vi "Get Kalman Filter State.vi"(11 "Kalman Filter In":T2) -> (0 "Predicted Covariance":T1, 1 "Predicted State":T1, 2 "Current Covariance":T1, 3 "Current State":T1)   [LabVIEW 2020]
uses:
  ctl/Kalman Filter Instance.ctl
  <vilib>/Analysis/Matrix/Datatypes/RealMatrix.ctl
  ctl/Dynamical System Matrices.ctl
  <vilib>/Analysis/Matrix/NI_Matrix.lvlib
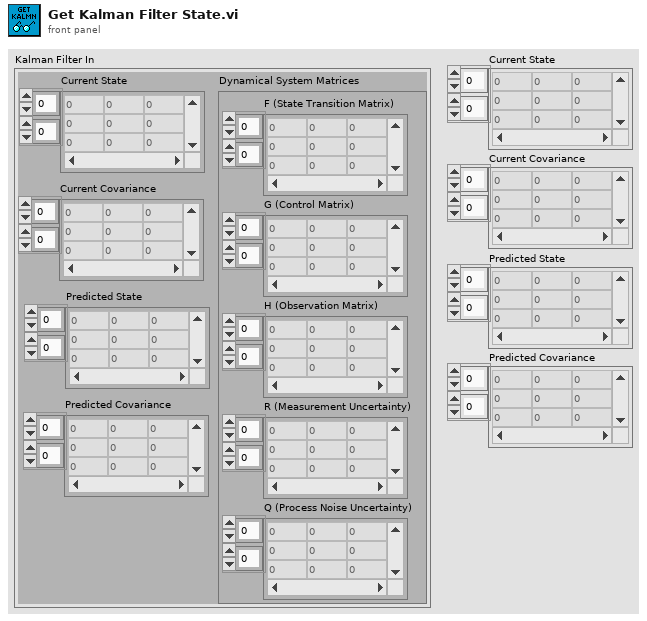
[diagram p1: front panel]
types:
  T1 = typedef "NI_Matrix.lvlib/RealMatrix.ctl" = dbl[][]
  T2 = typedef "Kalman Filter Instance.ctl" = cluster{"Current State":T1, "Current Covariance":T1, "Predicted State":T1, "Predicted Covariance":T1, "Dynamical System Matrices":T3}
  T3 = typedef "Dynamical System Matrices.ctl" = cluster{"F (State Transition Matrix)":T1, "G (Control Matrix)":T1, "H (Observation Matrix)":T1, "R (Measurement Uncertainty)":T1, "Q (Process Noise Uncertainty)":T1}
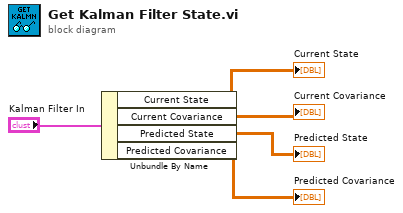
[diagram p0: block diagram]
diagram:
  n1 = Unbundle By Name("Kalman Filter In") -> ("Current State"=→"Current State":T1, "Current Covariance"=→"Current Covariance":T1, "Predicted State"=→"Predicted State":T1, "Predicted Covariance"=→"Predicted Covariance":T1)
